vi "Hidden Front.vi"(8 "error in (no error)":errorcluster, 11 "Abstruct View in":refnum<class "Abstruct View.lvclass">) -> (0 "error out":errorcluster, 3 "Abstruct View out":refnum<class "Abstruct View.lvclass">)   [LabVIEW 2020, in "Abstruct View.lvlib" / "Abstruct View.lvclass"]
uses:
  Abstruct View.lvclass
  Abstruct View.lvclass/Abstruct View.ctl
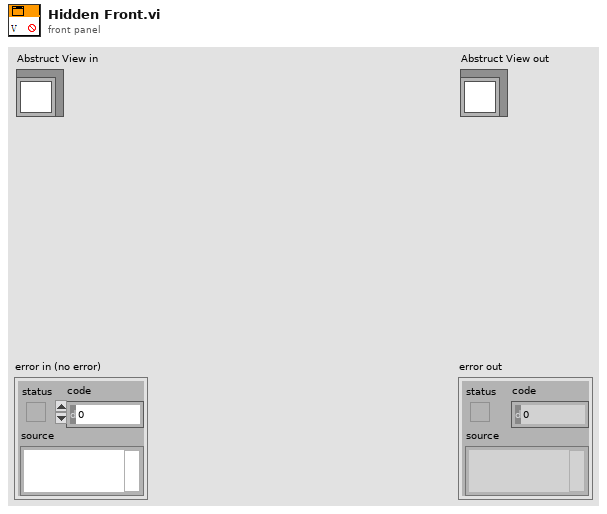
[diagram p1: front panel]
types:
  T1 = enum32{"Invalid", "Standard", "Closed", "Hidden", "Minimized", "Maximized"}
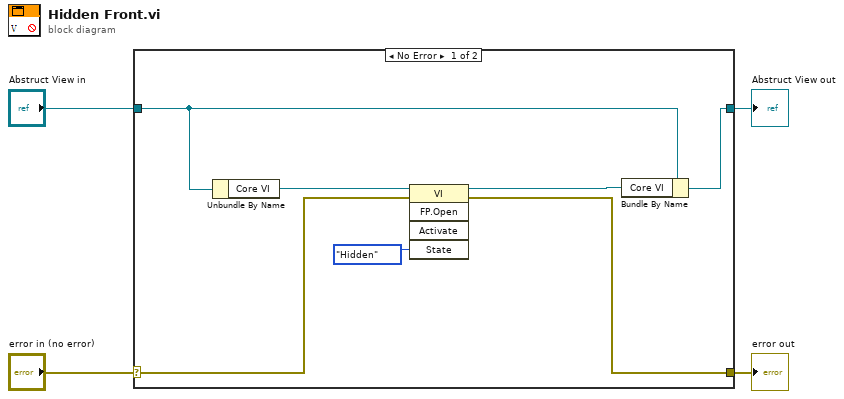
[diagram p0: block diagram]
diagram:
  n1 = case shown="No Error" "error in (no error)" {
    selector: "error in (no error)" -> [w7 w13]
    tunnel: [w6 w13] -> w3
    tunnel: [w5 w12] -> w1
    tunnel: "Abstruct View in" -> [w9 w12]
    frame No Error {
      n2 = Unbundle By Name(w9) -> ("Core VI"=w10:refnum<vi>)
      n3 = invoke class="VI" method="FP.Open"(reference=w10, error in=w7, "State"=T1."Hidden") -> (reference out=w8:refnum<vi>, error out=w6:errorcluster)  [unwired: 2 in, 3 out]
      n4 = Bundle By Name(cluster=w9, "Core VI"=w8) -> (w5:refnum<class "Abstruct View.lvclass">)
    }
    frame Error {
    }
  }
  "error out" <- w3
  "Abstruct View out" <- w1
